vi "Set Control Visibility.vi"(8 "Error in":errorcluster, 10 "States of Controls":bool[](array[boolean]), 11 "State Variables in":T1={"Stop Notifier"=refnum, "UI References"=[], "DAQmx"={"ECG Input"={"Channel"="", "Task"="", "Max Value"=0.0, "Min Value"=0.0, "Sampling Rate"=0.0, "Batch Size"=10}, "Trigger Output"={"Channel"="", "Task"="", "Pulse Frequency"=0.0, "Delay"=0, "Triggers per Shot"=0}}, "Data Queue"=refnum, "Filter"={"Batch Size"=1000, "Update Cycle"=0, "Filter Buffer"=[]}, "Last Detect Result"=FALSE}) -> (0 "Error out":errorcluster, 3 "State Variables out":T1={"Stop Notifier"=refnum, "UI References"=[], "DAQmx"={"ECG Input"={"Channel"="", "Task"="", "Max Value"=0.0, "Min Value"=0.0, "Sampling Rate"=0.0, "Batch Size"=10}, "Trigger Output"={"Channel"="", "Task"="", "Pulse Frequency"=0.0, "Delay"=0, "Triggers per Shot"=0}}, "Data Queue"=refnum, "Filter"={"Batch Size"=1000, "Update Cycle"=0, "Filter Buffer"=[]}, "Last Detect Result"=FALSE})   [LabVIEW 2014, in "Flow Control.lvlib"]
uses:
  Flow Control.lvlib
  Controls/State Variables.ctl
  Controls/DAQmx Variables.ctl
  Controls/Filter Variables.ctl
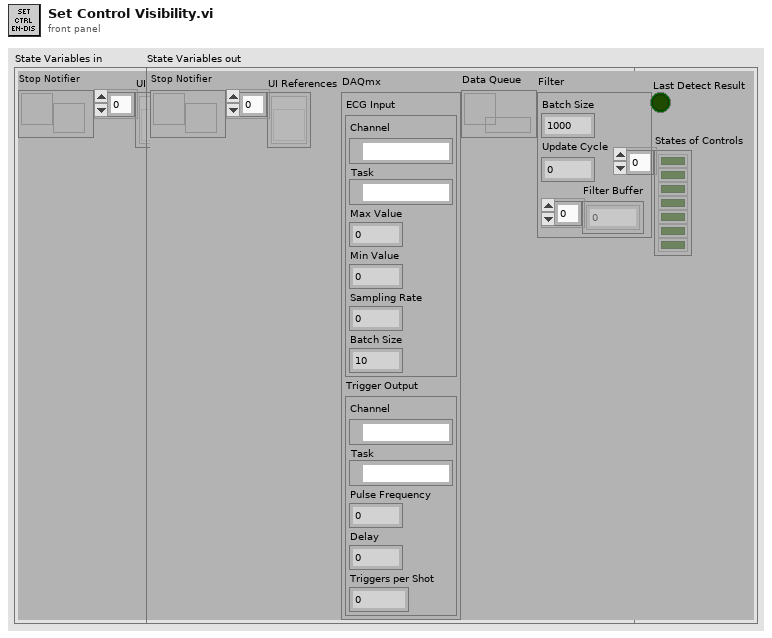
[diagram p1: front panel]
types:
  T1 = typedef "State Variables.ctl" = cluster{"Stop Notifier":refnum<notifier>, "UI References":refnum<vi>[], "DAQmx":T2, "Data Queue":refnum<queue>, "Filter":T3, "Last Detect Result":bool}
  T2 = typedef "DAQmx Variables.ctl" = cluster{"ECG Input":cluster{"Channel":tag, "Task":refnum<k21>, "Max Value":dbl, "Min Value":dbl, "Sampling Rate":dbl, "Batch Size":i32}, "Trigger Output":cluster{"Channel":tag, "Task":refnum<k21>, "Pulse Frequency":dbl, "Delay":u16, "Triggers per Shot":i32}}
  T3 = typedef "Filter Variables.ctl" = cluster{"Batch Size":i32, "Update Cycle":i32, "Filter Buffer":dbl[]}
  T4 = enum8{"Enabled", "Disabled", "Disabled and Grayed Out"}
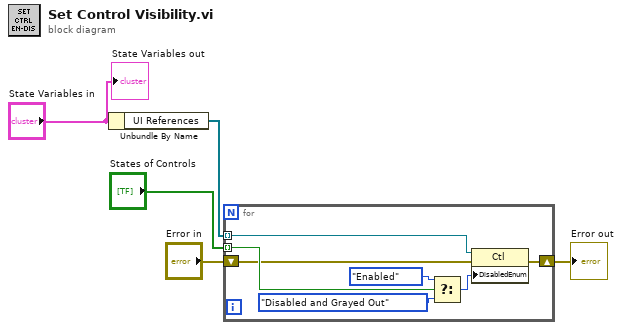
[diagram p0: block diagram]
diagram:
  n1 = Unbundle By Name("State Variables in") -> ("UI References"=w4:refnum<vi>[])
  n2 = for {
    tunnel: w4 -> [w12] mode=indexing
    tunnel: "States of Controls" -> [w10] mode=indexing
    shift-right: [w6] -> w1
    shift-left: "Error in" -> [w7]
    n3 = Select(t=T4."Enabled" ("Disabled"), s=w10, f=T4."Disabled and Grayed Out") -> (s? t:f=w8:T4)
    n4 = property class="Ctl"(reference=w12, error in=w7, "DisabledEnum"=w8) -> (error out=w6:errorcluster)  [unwired: 1 out]
  }
  "Error out" <- w1
  "State Variables out" <- "State Variables in"
